vi "Update Select Module Ring.vi"(8 "error in (no error)":errorcluster, 11 "Select Module Ring Ref":refnum<vi>) -> (0 "error out":errorcluster, 2 "Active Modules (Array)":string[](array[string]), 3 "New Module Ring Value":i32=-1)   [LabVIEW 2014, in "GenNet-Client.lvlib"]
doc: "Retrieve all currently running cloneable module instances and populate the module selector ring with their names and values.\n_____\nBased on Delacor QMH Project Template 3.1.0.34."
uses:
  GenNet-Client.lvlib
  Clone Registration/Clone Registration.lvlib
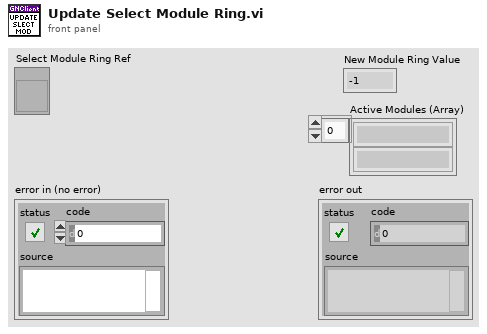
[diagram p1: front panel]
types:
  T1 = typedef "LVStringsAndValuesArrayTypeDef_I32.ctl" = cluster{"String":string, "Value":i32}[]
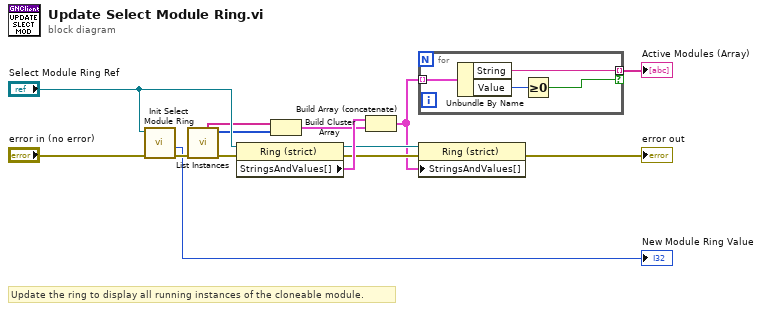
[diagram p0: block diagram]
diagram:
  # "Update the ring to display all running instances of the cloneable module."
  n1 = call "Init Select Module Ring.vi"("error in (no error)"="error in (no error)", "Select Module Ring Ref"="Select Module Ring Ref") -> ("error out"=w8:errorcluster, "Module Ring Value"=→"New Module Ring Value":i32)  [unwired: 7 in, 1 out]
  n2 = call "List Instances.vi"("error in (no error)"=w8) -> ("error out"=w14:errorcluster, "Module IDs"=w6:i32[], "Instances Names"=w7:string[])  [unwired: 6 in, 2 out]
  n3 = property on="Property Node" class="Ring (strict)"(reference="Select Module Ring Ref", error in=w14) -> (reference out=w10:refnum<vi>, error out=w11:errorcluster, "StringsAndValues[]"=w13:T1)
  n4 = Build Cluster Array(w7, w6) -> (w12:cluster{string, "Module ID":i32}[])
  n5 = Build Array (concatenate)(w13, w12) -> (w3:T1)
  n6 = for {
    tunnel: w3 -> [w18] mode=indexing
    tunnel: [w16] -> w2 mode=indexing if=w15
    n7 = Unbundle By Name(w18) -> ("String"=w16:string, "Value"=w17:i32)
    n8 = Greater Or Equal To 0?(x=w17) -> (x >= 0?=w15:bool)
  }
  "Active Modules (Array)" <- w2
  n9 = property on="Property Node" class="Ring (strict)"(reference=w10, error in=w11, "StringsAndValues[]"=w3) -> (error out=→"error out":errorcluster)  [unwired: 1 out]
